vi "Group Status.vi"(4 "Log Group":T1) -> (6 "Group Status":T4, 7 "Group":T1)   [LabVIEW 2020, in "VolatusGUIElements.lvlib" / "GroupLoggingControl.lvclass"]
uses:
  GroupLoggingControl.lvclass
  GroupLoggingControl.lvclass/GroupLoggingControl.ctl
  Log Group Status.ctl
  Command Info.ctl
  Log Group.ctl
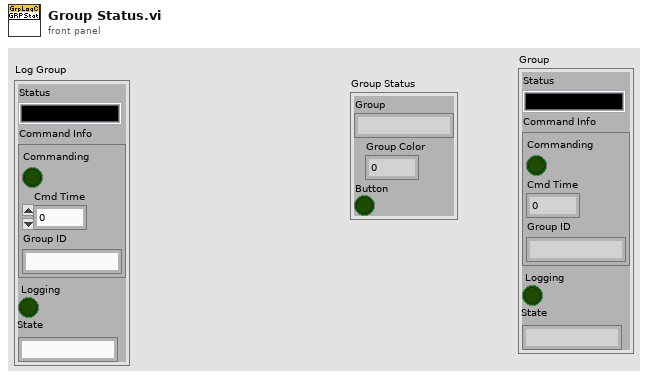
[diagram p1: front panel]
types:
  T1 = typedef "VolatusGUIElements.lvlib/GroupLoggingControl.lvclass/Log Group.ctl" = cluster{"Status":T2, "Command Info":T3, "Logging":bool, "State":string}
  T2 = typedef "VolatusGUIElements.lvlib/GroupLoggingControl.lvclass/Log Group Status.ctl" = cluster{"Group":string, "Group Color":u32, "Button":bool}
  T3 = typedef "VolatusGUIElements.lvlib/GroupLoggingControl.lvclass/Command Info.ctl" = cluster{"Commanding":bool, "Cmd Time":dbl, "Group ID":string}
  T4 = cluster{"Group":string, "Group Color":u32, "Button":bool}
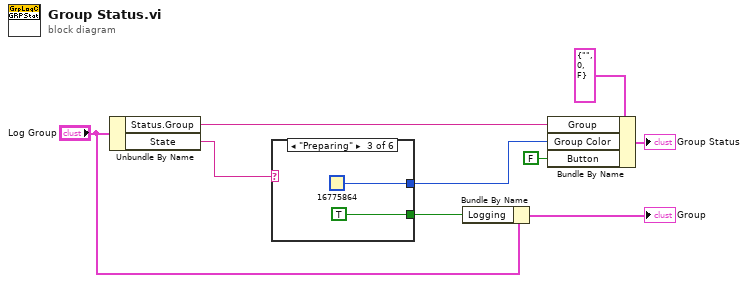
[diagram p0: block diagram]
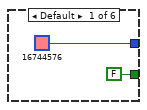
[diagram p2: hidden frame]
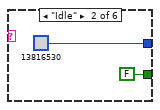
[diagram p3: hidden frame]
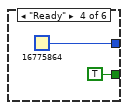
[diagram p4: hidden frame]
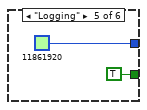
[diagram p5: hidden frame]
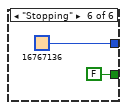
[diagram p6: hidden frame]
diagram:
  n1 = Unbundle By Name("Log Group") -> ("Status.Group"=w8:string, "State"=w1:string)
  n2 = case shown="\"Preparing\"" w1 {
    tunnel: [u32 16744576 u32 13816530 u32 16775864 u32 16775864 u32 11861920 u32 16767136] -> w6
    tunnel: [FALSE FALSE TRUE TRUE TRUE FALSE] -> w3
    frame Default {
    }
    frame "Idle" {
    }
    frame "Preparing" {
    }
    frame "Ready" {
    }
    frame "Logging" {
    }
    frame "Stopping" {
    }
  }
  n3 = Bundle By Name(cluster="Log Group", "Logging"=w3) -> (→"Group":T1)
  n4 = Bundle By Name(cluster=T4 {"Group"="", "Group Color"=0, "Button"=FALSE} ("Node Status 2"), "Group"=w8, "Group Color"=w6, "Button"=FALSE) -> (→"Group Status":T4)
